vi "EXA_putSample_loopTimeMs.vi"(8 "error in (no error)":errorcluster, 11 "loopTimeMs_Ctl":T1) -> (0 "error out":errorcluster, 2 "function return":i32, 3 "loopTimeMs_Ctl out":T1)   [LabVIEW 2016, in "SALLV_EXA.lvlib"]
doc: "int EXA_shm_putSample_loopTimeMsLV(EXA_loopTimeMsLV *loopTimeMs_Ctl );"
uses:
  SALLV_EXA.lvlib
  DataTypes/loopTimeMs.ctl
  SALLV_EXA.so
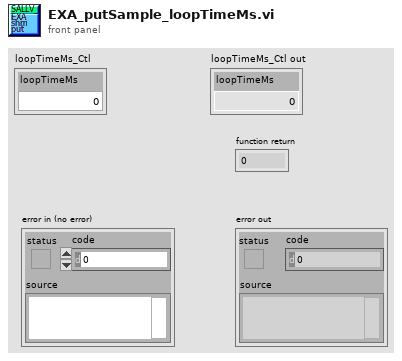
[diagram p1: front panel]
types:
  T1 = typedef "SALLV_EXA.lvlib/loopTimeMs.ctl" = cluster{"loopTimeMs":dbl}
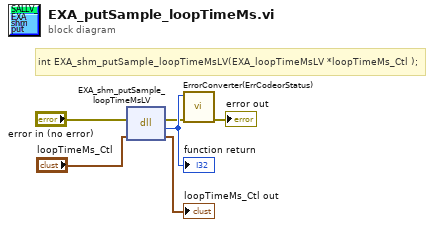
[diagram p0: block diagram]
diagram:
  # "int EXA_shm_putSample_loopTimeMsLV(EXA_loopTimeMsLV *loopTimeMs_Ctl );"
  n1 = dll-call lib="home/andres/Desktop/SAL_EXA/SALLV_EXA.*" fn="EXA_shm_putSample_loopTimeMsLV"(error in="error in (no error)", "loopTimeMs_Ctl"="loopTimeMs_Ctl") -> (error out=w2:errorcluster, w6:i32, "loopTimeMs_Ctl"=→"loopTimeMs_Ctl out":T1)  [unwired: 2 in, 1 out]
  "function return" <- w6
  n2 = call "ErrorConverter(ErrCodeorStatus).vi"("error in (no error)"=w2, "error code"=w6) -> ("error out"=→"error out":errorcluster)  [unwired: 9 in]
